vi "cmd_set_ao_gain.vi"(8 "error in (no error)":errorcluster, 11 "JSON":string) -> (0 "error out":errorcluster)   [LabVIEW 2021]
doc: "Sets the gain of the analogue input.\n\n :param gain: Specifies the ao gain (8ch)"
uses:
  core/host_global_vars.vi
  <vilib>/Utility/error.llb/Error Cluster From Error Code.vi
  <vilib>/rvi/errors/niLvFpgaAdjustHostInterfaceError.vi
  <vilib>/rvi/interface/nirviReadWriteControl/nirviReadWriteControl.xnode
  fpga/fpga_dtype_sgl_8ch.ctl
  FPGA Bitfiles/openlabspm_FPGATarget_fpgamain_eo-gUZR5D1g.lvbitx
  fpga/fpga_main.vi
  NiFpgaLv.dll
panel:
  in  "args":cluster{"gain":sgl[]}
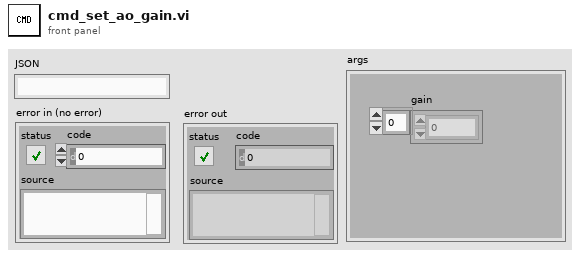
[diagram p1: front panel]
types:
  T1 = cluster{"gain[0]":sgl, "gain[1]":sgl, "gain[2]":sgl, "gain[3]":sgl, "gain[4]":sgl, "gain[5]":sgl, "gain[6]":sgl, "gain[7]":sgl}
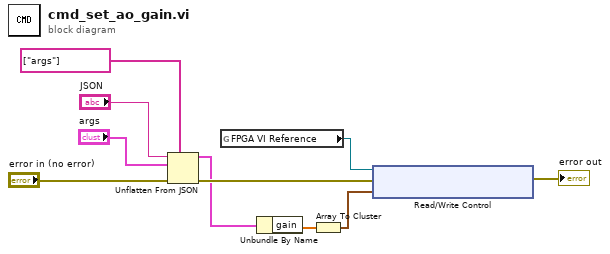
[diagram p0: block diagram]
diagram:
  n1 = Unflatten From JSON(path=string[] ["args"], JSON string="JSON", type and defaults="args", error in (no error)="error in (no error)") -> (value=w4:cluster{"gain":sgl[]}, error out=w5:errorcluster)  [unwired: 3 in]
  n2 = global read "host_global_vars.vi" "FPGA VI Reference"() -> (w6:refnum<k20>)
  n3 = Unbundle By Name(w4) -> ("gain"=w2:sgl[])
  n4 = Array To Cluster(array=w2) -> (cluster=w1:T1)
  n5 = xnode "Read/Write Control"("FPGA VI Reference In"=w6, "error in"=w5, "ao gain"=w1) -> ("error out"=→"error out":errorcluster)  [unwired: 1 out]
